vi "NI General Camera.vi"(4 "Camera Notifiers":T3, 6 "Refnums":T1, 8 "error in (no error)":errorcluster, 10 "Camera Name":refnum<k21> caption="IMAQdx Session", 11 "Function":T5) -> (0 "error out":errorcluster, 1 "Buffer Number":u32, 2 "Image":T4(plugin-control), 3 "Frame Rate":dbl)   [LabVIEW 2014]
uses:
  NI Camera Functions.ctl
  Camera Notifiers.ctl
  support/Instrument Status.ctl
  Camera Refnums.ctl
  support/Instrument Status State.ctl
  <vilib>/vision/driver/NI_Vision_Acquisition_Software.lvlib
panel:
  out "Instrument Status":T2
  # "LICENSED MATERIALS – PROPERTY OF IBM\nCopyright IBM Corp. 2016,\nALL RIGHTS RESERVED"
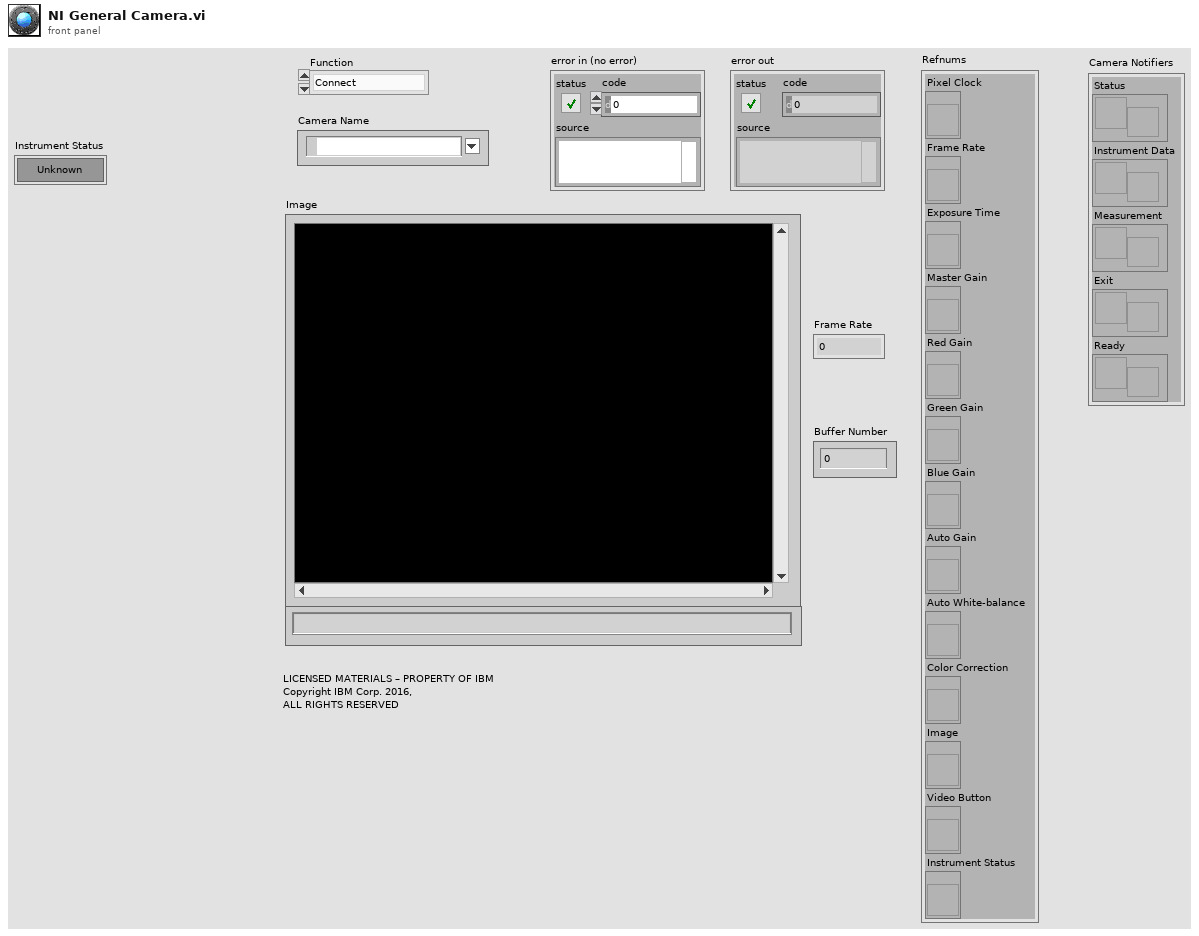
[diagram p1: front panel]
types:
  T1 = typedef "Camera Refnums.ctl" = cluster{"Pixel Clock":refnum<vi>, "Frame Rate":refnum<vi>, "Exposure Time":refnum<vi>, "Master Gain":refnum<vi>, "Red Gain":refnum<vi>, "Green Gain":refnum<vi>, "Blue Gain":refnum<vi>, "Auto Gain":refnum<vi>, "Auto White-balance":refnum<vi>, "Color Correction":refnum<vi>, "Image":refnum<vi>, "Video Button":refnum<vi>, "Instrument Status":refnum<vi>}
  T2 = typedef "Instrument Status.ctl" = bool
  T3 = typedef "Camera Notifiers.ctl" = cluster{"Status":refnum<notifier>, "Instrument Data":refnum<notifier>, "Measurement":refnum<notifier>, "Exit":refnum<notifier>, "Ready":refnum<notifier>}
  T4 = typedef "IMAQ Image.ctl" = refnum<image>
  T5 = typedef "NI Camera Functions.ctl" = enum16{"Connect", "Disconnect", "Start Live", "Stop Live", "Acquire", "Update Refnums"}
  T6 = typedef "Instrument Status State.ctl" = enum16{"Unknown", "Idle", "Standby", "Configuring", "Measuring", "Moving", "Disconnected"}
  T7 = typedef "IMAQdx.ctl" = refnum<k21>
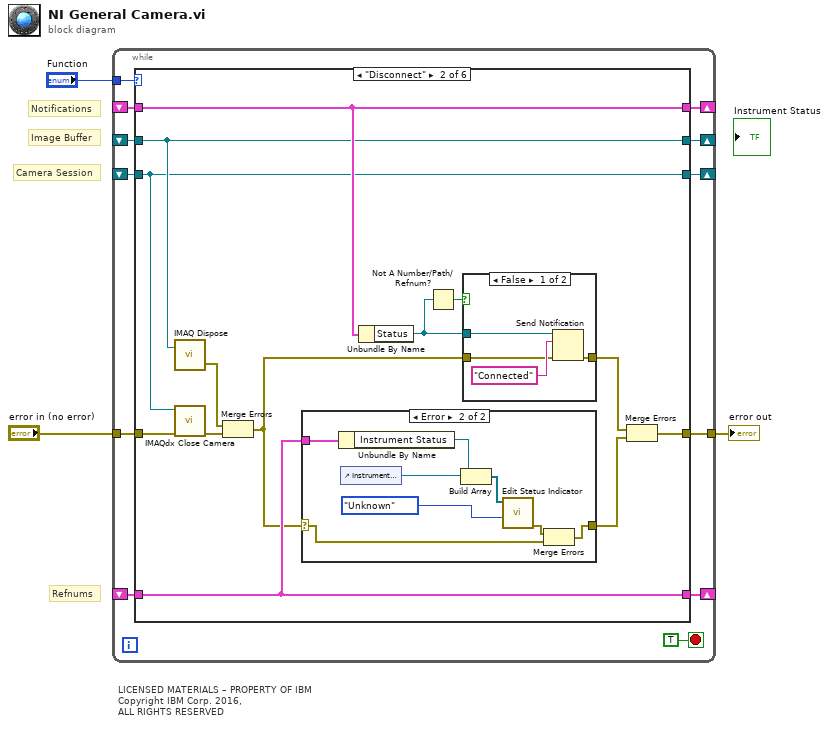
[diagram p0: block diagram]
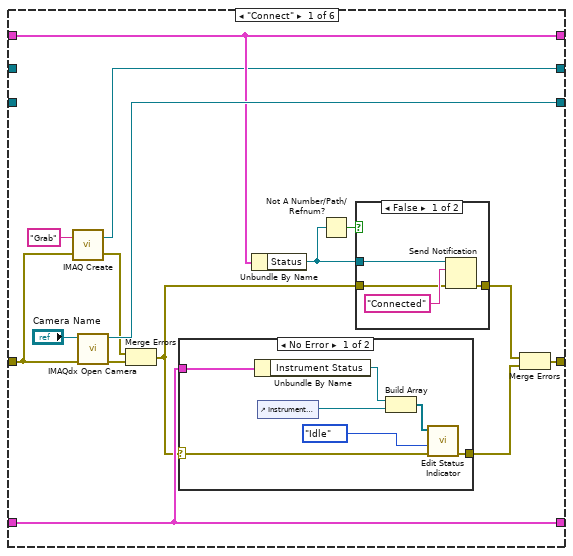
[diagram p2: hidden frame]
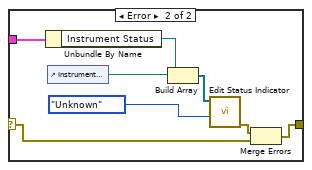
[diagram p3: hidden frame]
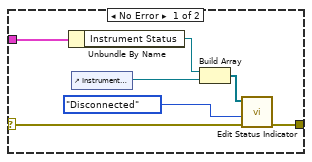
[diagram p5: hidden frame]
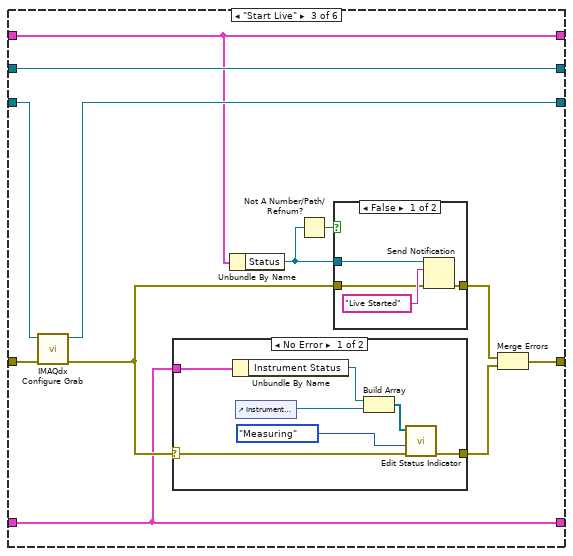
[diagram p7: hidden frame]
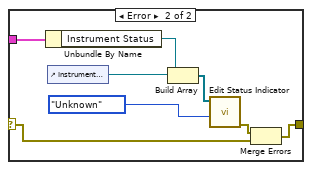
[diagram p8: hidden frame]
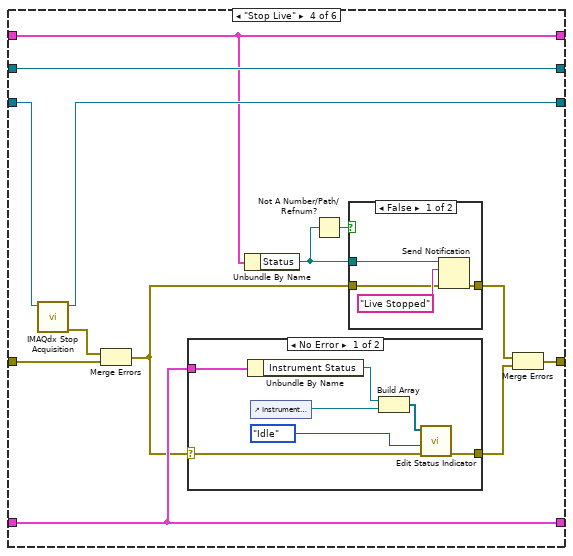
[diagram p10: hidden frame]
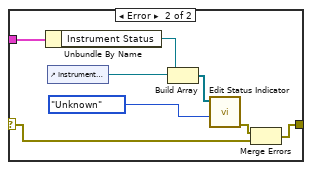
[diagram p11: hidden frame]
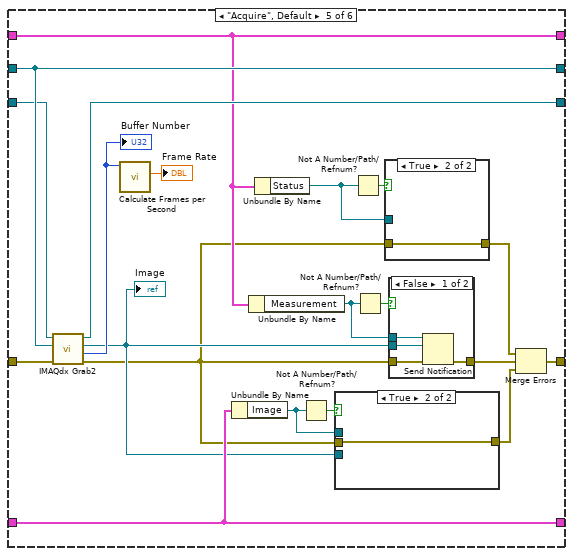
[diagram p13: hidden frame]
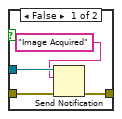
[diagram p14: hidden frame]
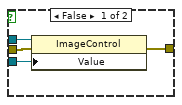
[diagram p16: hidden frame]
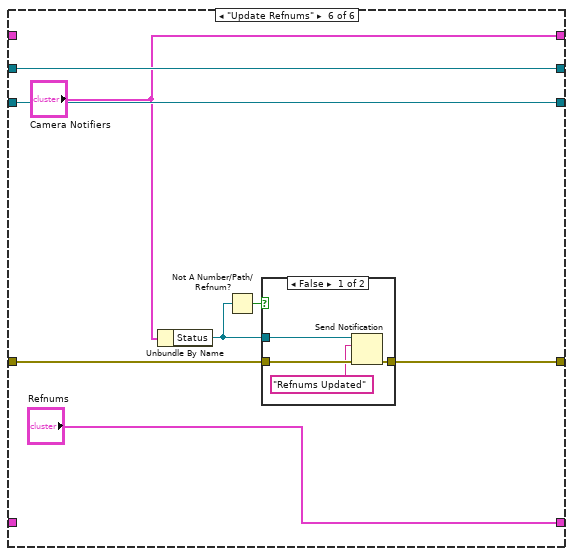
[diagram p17: hidden frame]
diagram:
  # "LICENSED MATERIALS – PROPERTY OF IBM\nCopyright IBM Corp. 2016,\nALL RIGHTS RESERVED"
  # "Notifications"
  # "Refnums"
  # "Camera Session"
  # "Image Buffer"
  n1 = while {
    tunnel: "Function" -> [w15]
    tunnel: [w14] -> w2
    tunnel: "error in (no error)" -> [w13]
    shift-right: [w12] -> _
    shift-left: _ -> [w11]
    shift-right: [w10] -> _
    shift-left: _ -> [w9]
    shift-right: [w6] -> _
    shift-left: _ -> [w7]
    shift-right: [w5] -> _
    shift-left: _ -> [w4]
    stop <- TRUE stop-if-true
    n2 = case shown="\"Disconnect\"" w15 {
      tunnel: [w23 w57 w86 w120 w159 w185] -> w14
      tunnel: w13 -> [w19 w63 w92 w116 w168 w186]
      tunnel: [w18 w54 w95 w128 w167 w191] -> w12
      tunnel: w11 -> [_ w54 w95 w128 w167 w191]
      tunnel: [w29 w51 w93 w126 w163 w190] -> w10
      tunnel: w9 -> [_ w51 w94 w127 w164 w190]
      tunnel: w7 -> [w21 w55 w85 w118 w160 _]
      tunnel: [w21 w55 w85 w118 w160 "Refnums"] -> w6
      tunnel: [w22 w56 w84 w119 w153 "Camera Notifiers"] -> w5
      tunnel: w4 -> [w22 w56 w84 w119 w153 _]
      frame "Connect" {
        n3 = call "IMAQ Create"("Image Name"="Grab", "error in (no error)"=w19) -> ("New Image"=w18:T4, "error out"=w16:errorcluster)  [unwired: 2 in, 1 out]
        n4 = call <vilib>:"IMAQdx Open Camera.vi"("error in"=w19, "Session In"="Camera Name") -> ("error out"=w24:errorcluster, "Session Out"=w29:T7)  [unwired: 1 in, 7 out]
        n5 = Merge Errors(w16, w24) -> (w17:errorcluster)
        n6 = case shown="No Error" w17 {
          selector: w17 -> [w36 w43]
          tunnel: [w35 w42] -> w25
          tunnel: w21 -> [w31 w39]
          frame No Error {
            n7 = Unbundle By Name(w31) -> ("Instrument Status"=w32:refnum<vi>)
            n8 = control-ref of="Instrument Status"() -> (w33:refnum<vi>)
            n9 = Build Array(w32, w33) -> (w34:refnum<vi>[])
            n10 = call "Edit Status Indicator.vi"("error in (no error)"=w36, "State"=Instrument_Status_State."Idle", "Instrument Status Refnum"=w34) -> ("error out"=w35:errorcluster)  [unwired: 1 in, 7 out]
          }
          frame Error {
            n11 = Unbundle By Name(w39) -> ("Instrument Status"=w38:refnum<vi>)
            n12 = control-ref of="Instrument Status"() -> (w40:refnum<vi>)
            n13 = Build Array(w38, w40) -> (w44:refnum<vi>[])
            n14 = call "Edit Status Indicator.vi"("State"=Instrument_Status_State."Unknown", "Instrument Status Refnum"=w44) -> ("error out"=w41:errorcluster)  [unwired: 2 in, 7 out]
            n15 = Merge Errors(w41, w43) -> (w42:errorcluster)
          }
        }
        n16 = Unbundle By Name(w22) -> ("Status"=w27:refnum<notifier>)
        n17 = Not A Number/Path/Refnum?(number/path/refnum=w27) -> (NaN/Path/Refnum?=w28:bool)
        n18 = case shown="False" w28 {
          tunnel: [w49 w50] -> w26
          tunnel: w27 -> [w48 _]
          tunnel: w17 -> [w46 w50]
          frame False {
            n19 = Send Notification(notification="Connected", notifier=w48, error in (no error)=w46) -> (error out=w49:errorcluster)  [unwired: 1 out]
          }
          frame True {
          }
        }
        n20 = Merge Errors(w26, w25) -> (w23:errorcluster)
      }
      frame "Disconnect" {
        n21 = call "IMAQ Dispose"("Image"=w54) -> ("error out"=w52:errorcluster)  [unwired: 5 in]
        n22 = call <vilib>:"IMAQdx Close Camera.vi"("error in"=w63, "Session In"=w51) -> ("error out"=w58:errorcluster)  [unwired: 9 out]
        n23 = Merge Errors(w52, w58) -> (w53:errorcluster)
        n24 = case shown="Error" w53 {
          selector: w53 -> [w69 w76]
          tunnel: [w68 w75] -> w59
          tunnel: w55 -> [w65 w72]
          frame No Error {
            n25 = Unbundle By Name(w65) -> ("Instrument Status"=w64:refnum<vi>)
            n26 = control-ref of="Instrument Status"() -> (w66:refnum<vi>)
            n27 = Build Array(w64, w66) -> (w67:refnum<vi>[])
            n28 = call "Edit Status Indicator.vi"("error in (no error)"=w69, "State"=Instrument_Status_State."Disconnected", "Instrument Status Refnum"=w67) -> ("error out"=w68:errorcluster)  [unwired: 1 in, 7 out]
          }
          frame Error {
            n29 = Unbundle By Name(w72) -> ("Instrument Status"=w71:refnum<vi>)
            n30 = control-ref of="Instrument Status"() -> (w73:refnum<vi>)
            n31 = Build Array(w71, w73) -> (w77:refnum<vi>[])
            n32 = call "Edit Status Indicator.vi"("State"=Instrument_Status_State."Unknown", "Instrument Status Refnum"=w77) -> ("error out"=w74:errorcluster)  [unwired: 2 in, 7 out]
            n33 = Merge Errors(w74, w76) -> (w75:errorcluster)
          }
        }
        n34 = Unbundle By Name(w56) -> ("Status"=w61:refnum<notifier>)
        n35 = Not A Number/Path/Refnum?(number/path/refnum=w61) -> (NaN/Path/Refnum?=w62:bool)
        n36 = case shown="False" w62 {
          tunnel: [w82 w83] -> w60
          tunnel: w61 -> [w81 _]
          tunnel: w53 -> [w79 w83]
          frame False {
            n37 = Send Notification(notification="Connected", notifier=w81, error in (no error)=w79) -> (error out=w82:errorcluster)  [unwired: 1 out]
          }
          frame True {
          }
        }
        n38 = Merge Errors(w60, w59) -> (w57:errorcluster)
      }
      frame "Start Live" {
        n39 = call <vilib>:"IMAQdx Configure Grab.vi"("error in"=w92, "Session In"=w94) -> ("error out"=w87:errorcluster, "Session Out"=w93:T7)  [unwired: 8 out]
        n40 = case shown="No Error" w87 {
          selector: w87 -> [w101 w108]
          tunnel: [w100 w107] -> w88
          tunnel: w85 -> [w97 w104]
          frame No Error {
            n41 = Unbundle By Name(w97) -> ("Instrument Status"=w96:refnum<vi>)
            n42 = control-ref of="Instrument Status"() -> (w98:refnum<vi>)
            n43 = Build Array(w96, w98) -> (w99:refnum<vi>[])
            n44 = call "Edit Status Indicator.vi"("error in (no error)"=w101, "State"=Instrument_Status_State."Measuring", "Instrument Status Refnum"=w99) -> ("error out"=w100:errorcluster)  [unwired: 1 in, 7 out]
          }
          frame Error {
            n45 = Unbundle By Name(w104) -> ("Instrument Status"=w103:refnum<vi>)
            n46 = control-ref of="Instrument Status"() -> (w105:refnum<vi>)
            n47 = Build Array(w103, w105) -> (w109:refnum<vi>[])
            n48 = call "Edit Status Indicator.vi"("State"=Instrument_Status_State."Unknown", "Instrument Status Refnum"=w109) -> ("error out"=w106:errorcluster)  [unwired: 2 in, 7 out]
            n49 = Merge Errors(w106, w108) -> (w107:errorcluster)
          }
        }
        n50 = Unbundle By Name(w84) -> ("Status"=w90:refnum<notifier>)
        n51 = Not A Number/Path/Refnum?(number/path/refnum=w90) -> (NaN/Path/Refnum?=w91:bool)
        n52 = case shown="False" w91 {
          tunnel: [w114 w115] -> w89
          tunnel: w90 -> [w113 _]
          tunnel: w87 -> [w111 w115]
          frame False {
            n53 = Send Notification(notification="Live Started", notifier=w113, error in (no error)=w111) -> (error out=w114:errorcluster)  [unwired: 1 out]
          }
          frame True {
          }
        }
        n54 = Merge Errors(w89, w88) -> (w86:errorcluster)
      }
      frame "Stop Live" {
        n55 = call <vilib>:"IMAQdx Stop Acquisition.vi"("Session In"=w127) -> ("error out"=w121:errorcluster, "Session Out"=w126:T7)  [unwired: 9 in]
        n56 = Merge Errors(w121, w116) -> (w117:errorcluster)
        n57 = case shown="No Error" w117 {
          selector: w117 -> [w134 w141]
          tunnel: [w133 w140] -> w122
          tunnel: w118 -> [w130 w137]
          frame No Error {
            n58 = Unbundle By Name(w130) -> ("Instrument Status"=w129:refnum<vi>)
            n59 = control-ref of="Instrument Status"() -> (w131:refnum<vi>)
            n60 = Build Array(w129, w131) -> (w132:refnum<vi>[])
            n61 = call "Edit Status Indicator.vi"("error in (no error)"=w134, "State"=Instrument_Status_State."Idle", "Instrument Status Refnum"=w132) -> ("error out"=w133:errorcluster)  [unwired: 1 in, 7 out]
          }
          frame Error {
            n62 = Unbundle By Name(w137) -> ("Instrument Status"=w136:refnum<vi>)
            n63 = control-ref of="Instrument Status"() -> (w138:refnum<vi>)
            n64 = Build Array(w136, w138) -> (w142:refnum<vi>[])
            n65 = call "Edit Status Indicator.vi"("State"=Instrument_Status_State."Unknown", "Instrument Status Refnum"=w142) -> ("error out"=w139:errorcluster)  [unwired: 2 in, 7 out]
            n66 = Merge Errors(w139, w141) -> (w140:errorcluster)
          }
        }
        n67 = Unbundle By Name(w119) -> ("Status"=w124:refnum<notifier>)
        n68 = Not A Number/Path/Refnum?(number/path/refnum=w124) -> (NaN/Path/Refnum?=w125:bool)
        n69 = case shown="False" w125 {
          tunnel: [w147 w148] -> w123
          tunnel: w124 -> [w146 _]
          tunnel: w117 -> [w144 w148]
          frame False {
            n70 = Send Notification(notification="Live Stopped", notifier=w146, error in (no error)=w144) -> (error out=w147:errorcluster)  [unwired: 1 out]
          }
          frame True {
          }
        }
        n71 = Merge Errors(w123, w122) -> (w120:errorcluster)
      }
      frame "Acquire", Default {
        n72 = call <vilib>:"IMAQdx Grab2.vi"("error in"=w168, "Image In"=w167, "Session In"=w164) -> ("error out"=w150:errorcluster, "Buffer Number Out"=w166:u32, "Image Out"=w151:T4, "Session Out"=w163:T7)  [unwired: 5 in]
        "Image" <- w151
        "Buffer Number" <- w166
        n73 = call <vilib>:"Calculate Frames per Second.vi"("Buffer Number"=w166) -> ("Processed Frames/s"=→"Frame Rate":dbl)  [unwired: 8 in, 2 out]
        n74 = Unbundle By Name(w160) -> ("Image"=w161:refnum<vi>)
        n75 = Unbundle By Name(w153) -> ("Measurement"=w154:refnum<notifier>)
        n76 = Unbundle By Name(w153) -> ("Status"=w157:refnum<notifier>)
        n77 = Not A Number/Path/Refnum?(number/path/refnum=w161) -> (NaN/Path/Refnum?=w162:bool)
        n78 = case shown="True" w162 {
          tunnel: [w182 w183] -> w158
          tunnel: w161 -> [w181 _]
          tunnel: w151 -> [w180 _]
          tunnel: w150 -> [w179 w183]
          frame False {
            n79 = property class="ImageControl"(reference=w181, error in=w179, "Value"=w180) -> (error out=w182:errorcluster)  [unwired: 1 out]
          }
          frame True {
          }
        }
        n80 = Not A Number/Path/Refnum?(number/path/refnum=w157) -> (NaN/Path/Refnum?=w156:bool)
        n81 = Not A Number/Path/Refnum?(number/path/refnum=w154) -> (NaN/Path/Refnum?=w155:bool)
        n82 = case shown="True" w156 {
          tunnel: [w172 w173] -> w149
          tunnel: w157 -> [w171 _]
          tunnel: w150 -> [w169 w173]
          frame False {
            n83 = Send Notification(notification="Image Acquired", notifier=w171, error in (no error)=w169) -> (error out=w172:errorcluster)  [unwired: 1 out]
          }
          frame True {
          }
        }
        n84 = case shown="False" w155 {
          tunnel: w150 -> [w177 w178]
          tunnel: [w176 w178] -> w152
          tunnel: w154 -> [w175 _]
          tunnel: w151 -> [w174 _]
          frame False {
            n85 = Send Notification(notification=w174, notifier=w175, error in (no error)=w177) -> (error out=w176:errorcluster)  [unwired: 1 out]
          }
          frame True {
          }
        }
        n86 = Merge Errors(w149, w152, w158) -> (w159:errorcluster)
      }
      frame "Update Refnums" {
        n87 = Unbundle By Name("Camera Notifiers") -> ("Status"=w188:refnum<notifier>)
        n88 = Not A Number/Path/Refnum?(number/path/refnum=w188) -> (NaN/Path/Refnum?=w187:bool)
        n89 = case shown="False" w187 {
          tunnel: w186 -> [w195 w196]
          tunnel: [w194 w196] -> w185
          tunnel: w188 -> [w193 _]
          frame False {
            n90 = Send Notification(notification="Refnums Updated", notifier=w193, error in (no error)=w195) -> (error out=w194:errorcluster)  [unwired: 1 out]
          }
          frame True {
          }
        }
      }
    }
  }
  "error out" <- w2
